vi "Copy Template.vi"(6 "Context":refnum<vi>, 8 "error in (no error)":errorcluster, 10 "Folder":path, 11 "Entity Name":string) -> (0 "error out":errorcluster, 3 "New Library Path":path)   [LabVIEW 2020, in "Conditum-Tools.lvlib" / "Entity Editor.lvclass"]
uses:
  Entity Editor.lvclass
  Entity Editor.lvclass/Entity Editor.ctl
  Conditum-Tools.lvlib
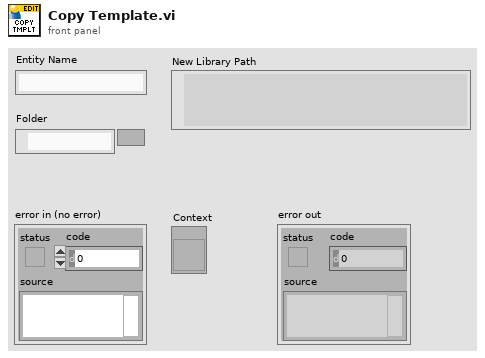
[diagram p1: front panel]
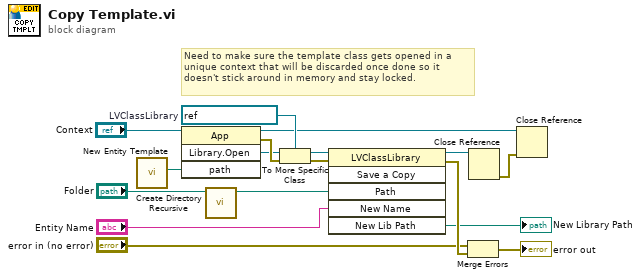
[diagram p0: block diagram]
diagram:
  w13 = refnum<vi> refnum  # LVClassLibrary
  # "Need to make sure the template class gets opened in a unique context that will be discarded once done so it doesn't stick around in memory and stay locked."
  n1 = call "New Entity Template.vi"() -> ("New Entity Template"=w2:path)  [unwired: 11 in]
  n2 = invoke class="App" method="Library.Open"(reference="Context", "path"=w2) -> (reference out=w3:refnum<vi>, error out=w16:errorcluster, "Open Library"=w14:refnum<vi>)  [unwired: 2 in, 1 out]
  n3 = call <vilib>:"Create Directory Recursive.vi"("directory"="Folder") -> ("directory copy"=w10:path)  [unwired: 4 in, 2 out]
  n4 = To More Specific Class(target class=w13, reference=w14, error in=w16) -> (specific class reference=w5:refnum<vi>, error out=w4:errorcluster)
  n5 = invoke class="LVClassLibrary" method="Save a Copy"(reference=w5, error in=w4, "Path"=w10, "New Name"="Entity Name") -> (reference out=w7:refnum<vi>, error out=w17:errorcluster, "New Lib Path"=→"New Library Path":path)  [unwired: 2 in, 3 out]
  n6 = Merge Errors("error in (no error)", w17) -> (→"error out":errorcluster)
  n7 = Close Reference(reference=w7) -> (error out=w6:errorcluster)  [unwired: 1 in]
  n8 = Close Reference(reference=w3, error in (no error)=w6) -> ()  [unwired: 1 out]
